vi "ReadHydDat.vi"(11 "Choose Directory":path) -> ()   [LabVIEW 2022 SP3]
uses:
  <vilib>/Math Plots/3D Math Plots/3D Waterfall/3D Waterfall Datatype/3D Waterfall Datatype.lvclass
  <vilib>/regexp/Match Regular Expression.xnode
  <vilib>/Math Plots/3D Math Plots/3D Waterfall/3D Waterfall Datatype/Public/Plot Helper (Vector).vi
  <vilib>/Utility/file.llb/Write To Spreadsheet File (DBL).vi
  <vilib>/Math Plots/3D Math Plots/3D Waterfall/3D Waterfall XCtrl/3D Waterfall.xctl
panel:
  out "Waveform Graph":dbl[](graph)
  in  "Boolean":bool
  out "3D Waterfall 2":refnum<class "3D Plot Datatype.lvclass">[](xcontrol)
  out "3D Waterfall":refnum<class "3D Plot Datatype.lvclass">[](xcontrol)
  in  "index (row)":i32
  in  "Use Selected Files":bool
  in  "Listbox":i32[](listbox)
  in  "file ext":string="eye"
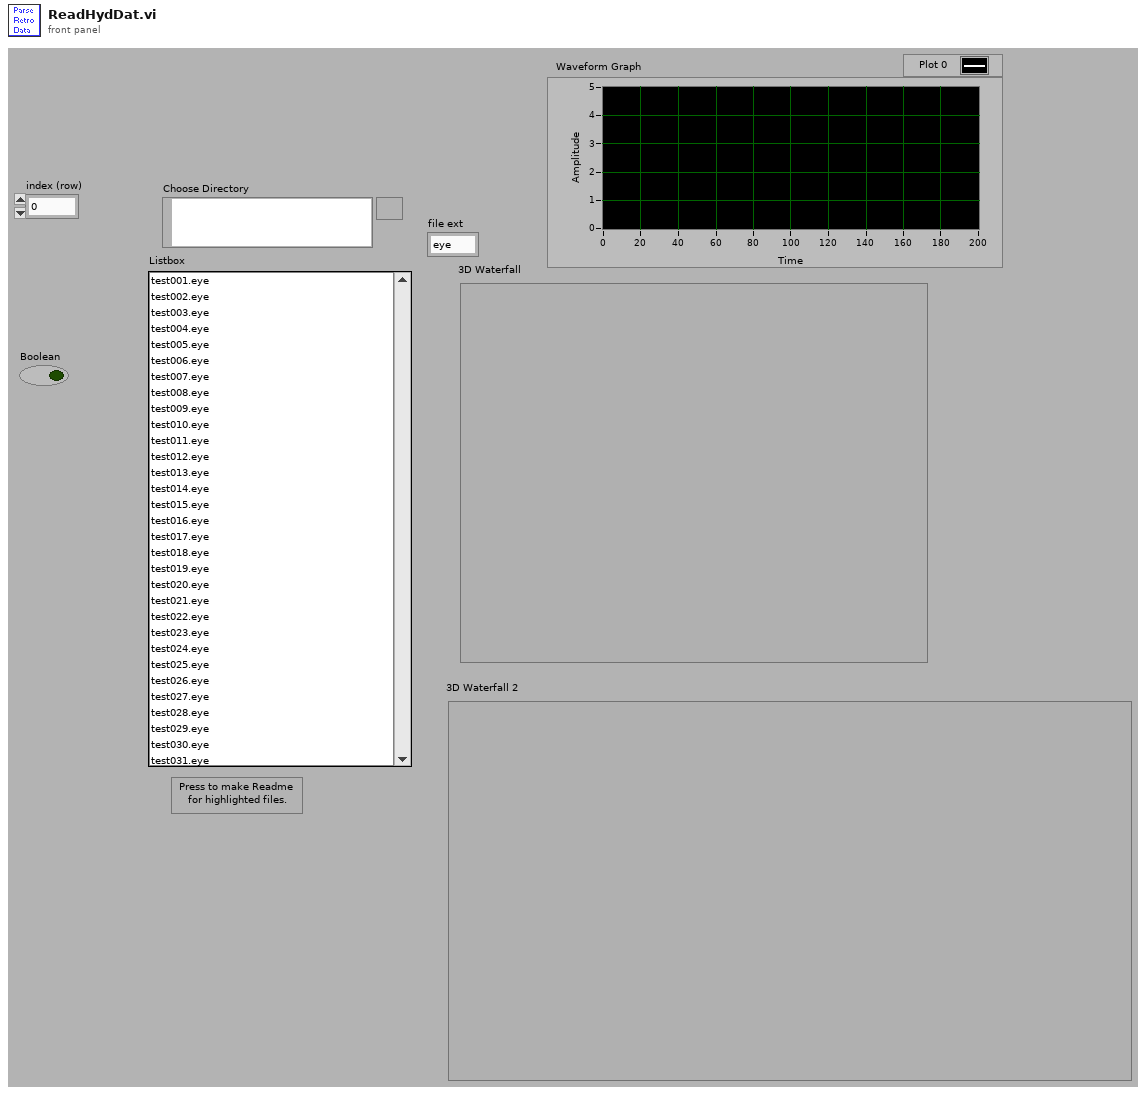
[diagram p1: front panel]
types:
  T1 = typedef "Header.ctl" = cluster{"header info":cluster{"Header":string, "Head length":i16}, "A/D info":cluster{"# rf points per line":u16, "# lines per scan":u16, "sample rate MHz":u16, "# A/D bits":i16, "# bytes per A/D":u16, "TGC Flag":u16, "A/D Type":string}, "Tranducer Info":cluster{"bandwidth":sgl, "center freq":sgl, "start freq":sgl, "ID":i32}, "Scan Info":cluster{"delay":sgl, "pivot distance":sgl, "sector scan angle":sgl, "operator":string, "Scan Mode":string, "location":string}, "Time/Date Info":cluster{"date":string, "time":string}, "RF Info":cluster{"RF file name":string, "RF file att":string, "RF cal file name":string, "RF cal file att":string}, "Patient Info":cluster{"ID":string, "extended ID":string, "age":u16, "sex":string, "previously\nscanned":string, "PSA":sgl, "LOS":u8, "Ethnicty 2":u8, "Race":u8}, "Tissue Type":cluster{"organ":i16, "disease type":i16, "disease location":i16, "IQ_pts":u16, "RcvBuffer":u8, "RcvFrame":u16, "IQBuff":u8, "IQFrame":u16, "IQPage":u8}, "Votage scaling":cluster{"Digitizer (dB)":sgl, "Gain (dB)":sgl, "Atten (dB)":sgl}, "Comment":string, "Misc Info":cluster{"avg num":u16, "c speed":i16, "Div By or SF zones":i16, "XMIT CHS":u8, "RCV CHS":u8, "Xmit angle":sgl}, "Therapy Parameters":cluster{"Theraputic Freq (MHz)":sgl, "Time on (s)":sgl, "Therapy amplitude (mV)":sgl, "Lines Before":u16, "Lines After":u16}, "Scan Settings":cluster{"Energy (uJ or V)":u8, "Damp (Ohm) or Fc":u8, "HP Filt (KHz)":u8, "LP Filt (MHz)":u8, "Gain (db)":u8, "prf (kHz)":sgl, "Distance between\nscan lines (um)":u16, "Distance between\nscan planes (um)":u16, "Scan line gap (um)":sgl, "Scan plane gap (um)":sgl}, "Compression Parameters":cluster{"F1 (MHz)":sgl, "F2 (MHz)":sgl, "% taper":sgl, "duration":sgl}, "Patient Info Xtra":cluster{"First Name":string, "Last Name":string, "Notes":string}, "ROI Box":u16[]}
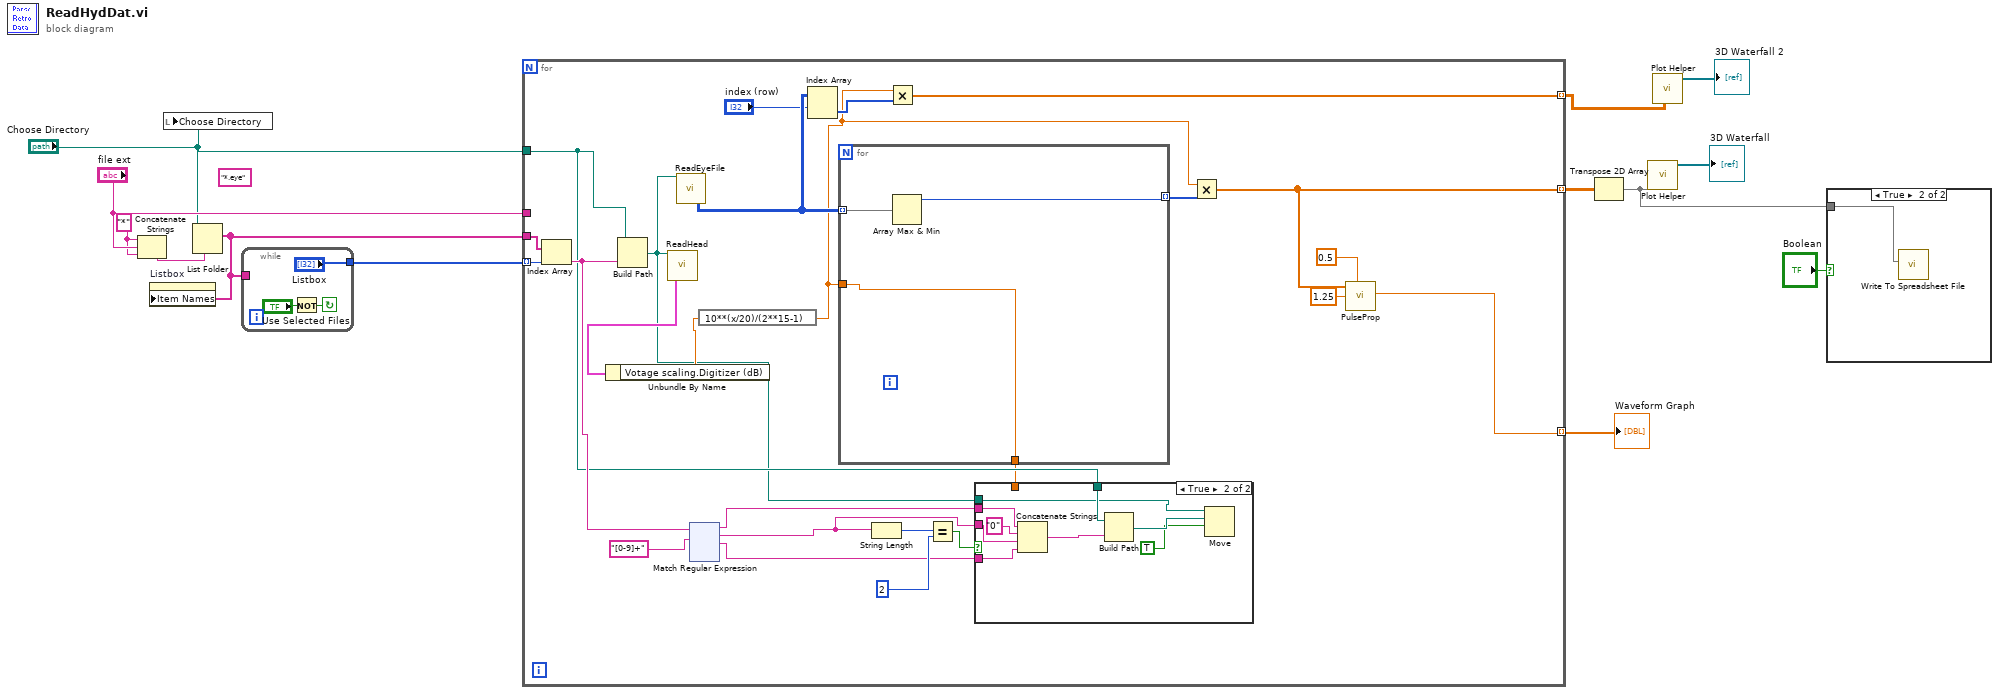
[diagram p0: block diagram]
diagram:
  w6 = "*" ("prompt")
  (unwired) "*.eye" ("prompt")
  n1 = Concatenate Strings(w6, "file ext", w6) -> (w7:string)
  n2 = local write "Choose Directory"("Choose Directory") -> ()
  n3 = List Folder(path="Choose Directory", pattern=w7) -> (filenames=w12:string[])  [unwired: 1 in, 4 out]
  n4 = property on="Listbox" class="LstBox (strict)"("Item Names"=w12) -> ()  [unwired: 2 in, 2 out]
  n5 = while {
    tunnel: ["Listbox"] -> w13
    tunnel: w12 -> [_]
    stop <- w16 continue-if-true
    n6 = Not(x="Use Selected Files") -> (.not. x?=w16:bool)
  }
  n7 = for {
    tunnel: w13 -> [w41] mode=indexing
    tunnel: w12 -> [w40]
    tunnel: "file ext" -> [_]
    tunnel: "Choose Directory" -> [w24]
    tunnel: [w34] -> w4 mode=indexing
    tunnel: [w20] -> w8 mode=indexing
    tunnel: [w17] -> w1 mode=indexing
    n8 = Index Array(array=w40, index=w41) -> (element=w29:string)
    n9 = Build Path(base path=w24, name or relative path=w29) -> (appended path=w23:path)
    n10 = call "ReadHead.vi"("new file path"=w23) -> ("Header In"=w39:T1)  [unwired: 18 out]
    n11 = Unbundle By Name(w39) -> ("Votage scaling.Digitizer (dB)"=w38:sgl)
    n12 = call "ReadEyeFile.vi"("new file path"=w23) -> ("2-D data array"=w37:i16[][])  [unwired: 1 in, 17 out]
    n13 = xnode "Match Regular Expression"("input string"=w29, "regular expression"="[0-9]+") -> ("before match"=w27:string, "whole match"=w25:string, "after match"=w26:string)  [unwired: 4 in, 2 out]
    n14 = expression code="10**(x/20)/(2**15-1)"(w38) -> (w22:sgl)
    n15 = Index Array(array=w37, index (row)="index (row)") -> (element=w35:i16[])  [unwired: 1 in]
    n16 = for {
      tunnel: w37 -> [w170] mode=indexing
      tunnel: [w169] -> w33 mode=indexing
      tunnel: w22 -> [w168]
      tunnel: [w168] -> w21
      n17 = Array Max & Min(array=w170) -> (max value=w169:i16)  [unwired: 3 out]
    }
    n18 = String Length(string=w25) -> (length=w31:i32)
    n19 = Multiply(x=w22, y=w35) -> (x*y=w34:sgl[])
    n20 = Equal?(x=w31, y=2) -> (x = y?=w28:bool)
    n21 = case shown="True" w28 {
      tunnel: w27 -> [_ w50]
      tunnel: w26 -> [_ w49]
      tunnel: w25 -> [_ w47]
      tunnel: w24 -> [_ w46]
      tunnel: w23 -> [_ w45]
      tunnel: w21 -> [_ _]
      frame False {
      }
      frame True {
        n22 = Concatenate Strings(w50, "0", w47, w49) -> (w42:string)
        n23 = Build Path(base path=w46, name or relative path=w42) -> (appended path=w44:path)
        n24 = Move(source path=w45, 9:TRUE ("overwrite (F)"), 10:w44) -> ()  [unwired: 2 in, 3 out]
      }
    }
    n25 = Multiply(x=w22, y=w33) -> (x*y=w20:sgl[])
    n26 = call "PulseProp.vi"("Data"=w20, "Scale factor"=0.5, "spacing"=1.25) -> ("width"=w17:dbl)  [unwired: 1 in, 6 out]
  }
  "Waveform Graph" <- w1
  n27 = Transpose 2D Array(2D array=w8) -> (transposed array=w3:sgl[][])
  n28 = call-poly <vilib>:"Plot Helper.vi"("z matrix"=w3) -> ("3D Plot lvclass Array out"=→"3D Waterfall":refnum<class "3D Plot Datatype.lvclass">[])  [unwired: 5 in, 5 out]
  n29 = call-poly <vilib>:"Plot Helper.vi"("z matrix"=w4) -> ("3D Plot lvclass Array out"=→"3D Waterfall 2":refnum<class "3D Plot Datatype.lvclass">[])  [unwired: 5 in, 5 out]
  n30 = case shown="True" "Boolean" {
    tunnel: w3 -> [_ w171]
    frame False {
    }
    frame True {
      n31 = call-poly <vilib>:"Write To Spreadsheet File.vi"("2D data"=w171) -> ()  [unwired: 7 in, 1 out]
    }
  }
